vi "GE 5565PIORC.PIO.Read (I64).vi"(7 "byte order (big-endian)":T1(ring), 8 "error in (no error)":errorcluster, 10 "offset":u32, 11 "GE 5565PIORC in":refnum<class "GE 5565PIORC.lvclass">) -> (0 "error out":errorcluster, 1 "data":i64, 3 "GE 5565PIORC out":refnum<class "GE 5565PIORC.lvclass">)   [LabVIEW 2017, in "GE 5565PIORC.lvclass"]
doc: "Reads <B>data</B> from the specified <B>offset</B>."
uses:
  GE 5565PIORC.lvclass
  <vilib>/Instr/_visa.llb/VISA Register Access Address Space.ctl
  GE 5565PIORC.lvclass/GE 5565PIORC.ctl
  GE 5565PIORC.VISA.Move In.String (U8).vi
  GE 5565PIORC.VISA.Return Handler.vi
  <vilib>/Utility/error.llb/Error Cluster From Error Code.vi
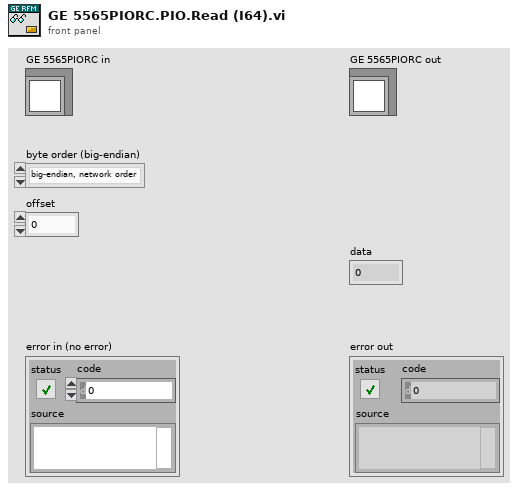
[diagram p1: front panel]
types:
  T1 = enum16{"big-endian, network order", "native, host order", "little-endian"}
  T2 = typedef "VISA Register Access Address Space.ctl" = u16
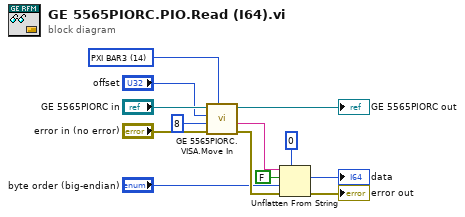
[diagram p0: block diagram]
diagram:
  w3 = T2 14 items=["VXI/VME A16"=1, "VXI/VME A24"=2, "VXI/VME A32"=3, "VXI/VME A64"=4, "PXI Memory Allocations"=9, "PXI Configuration"=10, "PXI BAR0"=11, "PXI BAR1"=12, "PXI BAR2"=13, "PXI BAR3"=14, "PXI BAR4"=15, "PXI BAR5"=16] ("address space")
  n1 = call-poly "GE 5565PIORC.VISA.Move In.vi"("address space"=w3, "error in (no error)"="error in (no error)", "count"=u32 8, "offset"="offset", "GE 5565PIORC in"="GE 5565PIORC in") -> ("error out"=w9:errorcluster, "data out"=w8:string, "GE 5565PIORC out"=→"GE 5565PIORC out":refnum<class "GE 5565PIORC.lvclass">)  [unwired: 4 in]
  n2 = Unflatten From String(type=i64 0, binary string=w8, data includes array or string size? (T)=FALSE, byte order (0:big-endian, network order)="byte order (big-endian)", error in (no error)=w9) -> (value=→"data":i64, error out=→"error out":errorcluster)  [unwired: 1 out]
